vi "Get sensor alert status.vi"(8 "Error In":errorcluster, 10 "MAC address":string) -> (0 "Error Out":errorcluster, 2 "Is Alert Active?":bool)   [LabVIEW 2016]
uses:
  <vilib>/Utility/file.llb/Read Delimited Spreadsheet (string).vi
  <vilib>/Utility/file.llb/Write Delimited Spreadsheet (string).vi
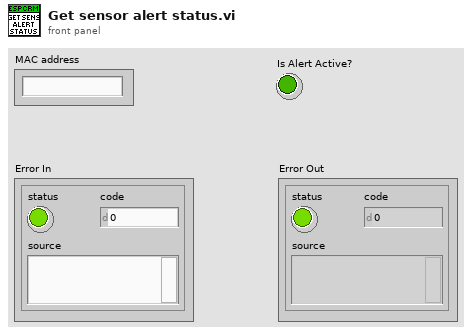
[diagram p1: front panel]
types:
  T1 = enum16{"open", "replace", "create", "open or create", "replace or create", "replace or create with confirmation"}
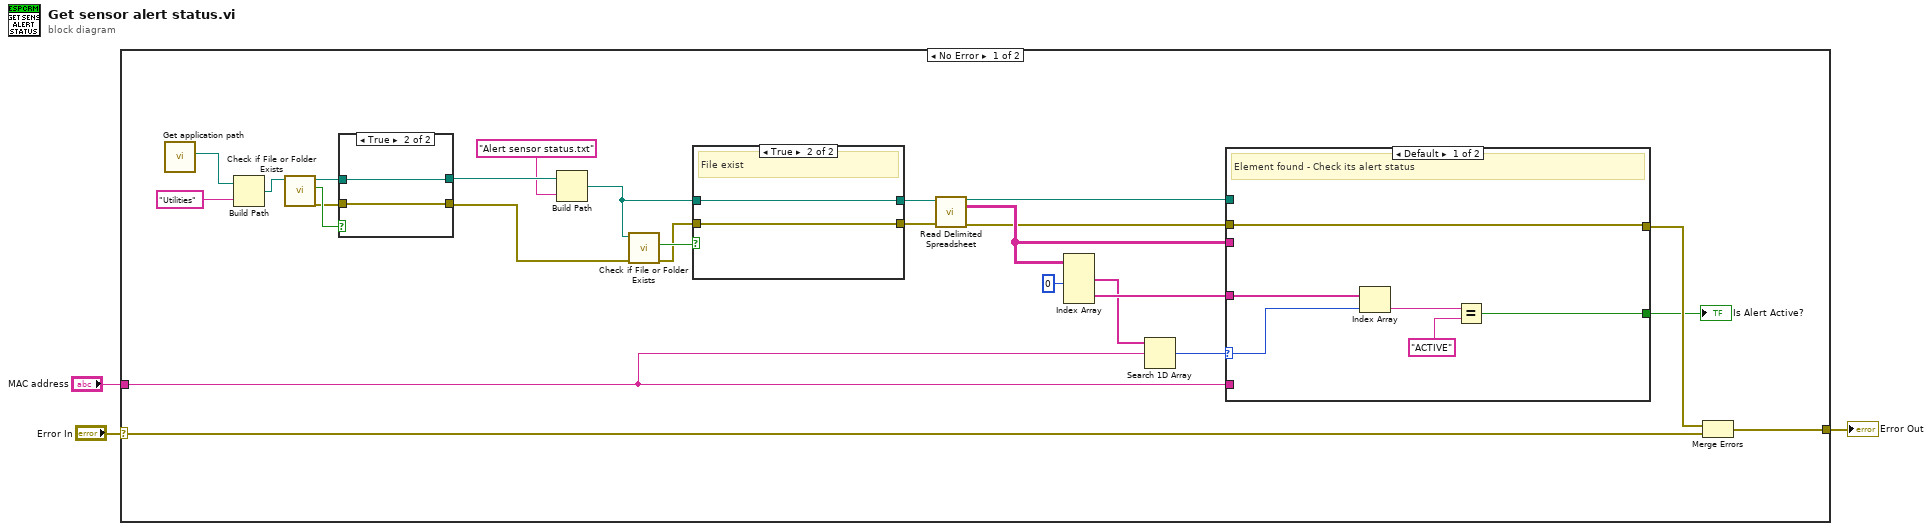
[diagram p0: block diagram]
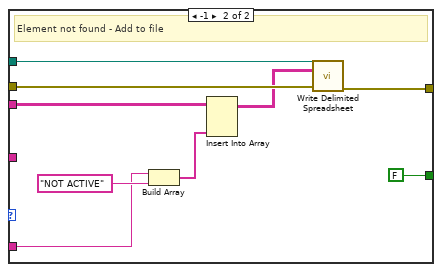
[diagram p2: hidden frame]
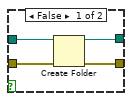
[diagram p3: hidden frame]
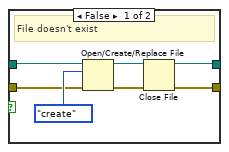
[diagram p4: hidden frame]
diagram:
  n1 = case shown="No Error" "Error In" {
    selector: "Error In" -> [w13 w60]
    tunnel: "MAC address" -> [w9 _]
    tunnel: [w12 w60] -> w1
    frame No Error {
      n2 = call "Get application path.vi"() -> ("Application path"=w20:path)  [unwired: 11 in]
      n3 = Build Path(base path=w20, name or relative path="Utilities") -> (appended path=w22:path)
      n4 = call <vilib>:"Check if File or Folder Exists.vi"("path"=w22) -> ("error out"=w26:errorcluster, "file or folder exists?"=w27:bool, "dup path"=w25:path)  [unwired: 8 in]
      n5 = case shown="True" w27 {
        tunnel: w26 -> [w48 w49]
        tunnel: w25 -> [w47 w50]
        tunnel: [w46 w50] -> w24
        tunnel: [w45 w49] -> w19
        frame False {
          n6 = Create Folder(path (use dialog)=w47, error in=w48) -> (created path=w46:path, error out=w45:errorcluster)  [unwired: 1 in, 1 out]
        }
        frame True {
        }
      }
      n7 = Build Path(base path=w24, name or relative path="Alert sensor status.txt") -> (appended path=w28:path)
      n8 = call <vilib>:"Check if File or Folder Exists.vi"("error in (no error)"=w19, "path"=w28) -> ("error out"=w18:errorcluster, "file or folder exists?"=w29:bool)  [unwired: 7 in, 1 out]
      n9 = case shown="True" w29 {
        tunnel: [w54 w59] -> w16
        tunnel: w28 -> [w53 w59]
        tunnel: w18 -> [w52 w58]
        tunnel: [w51 w58] -> w14
        frame False {
          # "File doesn't exist"
          n10 = Open/Create/Replace File(file path (use dialog)=w53, error in=w52, operation (0:open)=T1."create") -> (refnum out=w55:refnum<file>, error out=w56:errorcluster)  [unwired: 3 in, 1 out]
          n11 = Close File(refnum=w55, error in=w56) -> (path=w54:path, error out=w51:errorcluster)
        }
        frame True {
          # "File exist"
        }
      }
      n12 = call-poly <vilib>:"Read Delimited Spreadsheet.vi"("file path (dialog if empty)"=w16, "error in (no error)"=w14) -> ("new file path (Not A Path if cancelled)"=w7:path, "all rows"=w8:string[][], "error out"=w6:errorcluster)  [unwired: 8 in, 3 out]
      n13 = Index Array(array=w8, index (col) #1=0 ("disabled index (col)")) -> (element #1=w10:string[], element #2=w15:string[])  [unwired: 3 in]
      n14 = Search 1D Array(1D array=w10, element=w9) -> (index of element=w11:i32)  [unwired: 1 in]
      n15 = case shown="Default" w11 {
        selector: w11 -> [w32 _]
        tunnel: w15 -> [w35 _]
        tunnel: w9 -> [_ w42]
        tunnel: w8 -> [_ w44]
        tunnel: w7 -> [_ w40]
        tunnel: w6 -> [w31 w39]
        tunnel: [w31 w38] -> w5
        tunnel: [w30 FALSE] -> w4
        frame Default {
          # "Element found - Check its alert status"
          n16 = Index Array(array=w35, index=w32) -> (element=w34:string)
          n17 = Equal?(x=w34, y="ACTIVE") -> (x = y?=w30:bool)
        }
        frame -1 {
          # "Element not found - Add to file"
          n18 = Build Array(w42, "NOT ACTIVE") -> (w41:string[])
          n19 = Insert Into Array(array=w44, new element=w41) -> (w37:string[][])  [unwired: 2 in]
          n20 = call-poly <vilib>:"Write Delimited Spreadsheet.vi"("file path (dialog if empty)"=w40, "2D data"=w37, "error in (no error)"=w39) -> ("error out"=w38:errorcluster)  [unwired: 11 in, 1 out]
        }
      }
      "Is Alert Active?" <- w4
      n21 = Merge Errors(w5, w13) -> (w12:errorcluster)
    }
    frame Error {
    }
  }
  "Error Out" <- w1
